vi "Equalize Channel.vi"(0 "input data":cdb[](array[numeric])=array[8192 elements], 7 "channel":T1) -> (3 "processing duration":dbl format="%#_6p", 4 "output data":cdb[](array[numeric]))   [LabVIEW 2019]
uses:
  3fdb30cd-5524-4ae9-8a8d-15974dc7fefb.vi
  <vilib>/Analysis/1siggen.llb/Ramp Pattern by Samples.vi
  <vilib>/Analysis/2dsp.llb/Complex FFT.vi
  <vilib>/Analysis/2dsp.llb/Inverse Complex FFT.vi
  e220b846-d6bb-41e5-8f9d-4ae727cf2950.vi
  <vilib>/Utility/High Resolution Relative Seconds.vi
  <vilib>/Utility/error.llb/Clear Errors.vi
  <vilib>/Analysis/NI_AALPro.lvlib
  <vilib>/Analysis/NI_AALBase.lvlib
  <vilib>/gmath/NI_Gmath.lvlib
panel:
  out "XY Graph":cluster{"xi used":dbl[], "yi":dbl[]}[](graph)
  out "XY Graph 2":cluster{"xi used":dbl[], "yi":dbl[]}(graph)
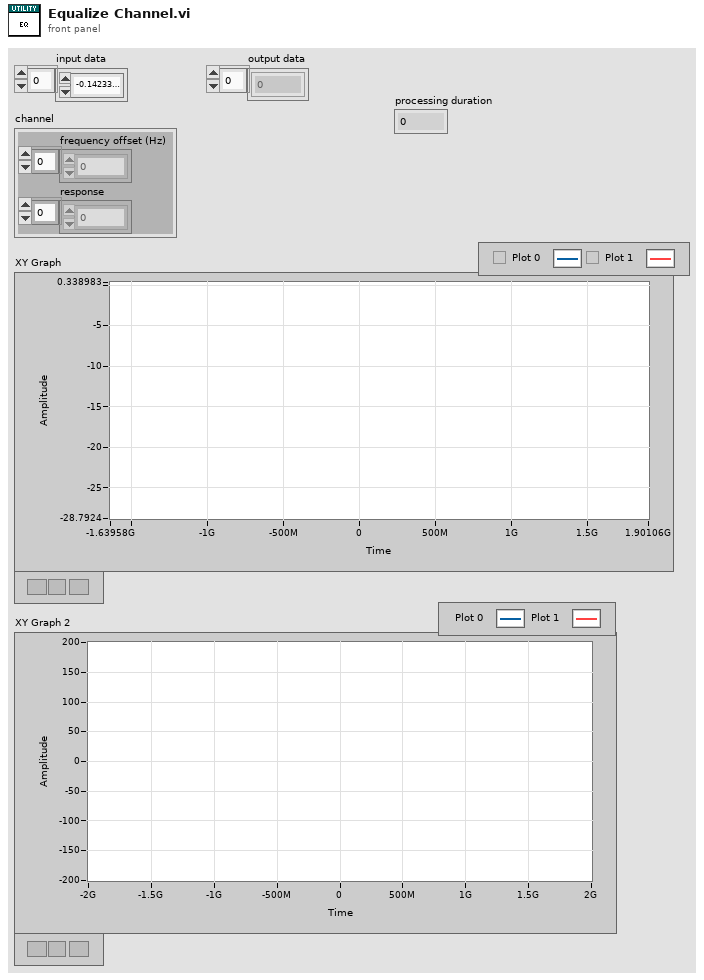
[diagram p1: front panel]
types:
  T1 = cluster{"frequency offset (Hz)":dbl[], "response":cdb[]}
  T2 = typedef "Constants.ctl" = cluster{"data clock rate (Hz)":dbl, "sample rate (Hz)":dbl, "sample rate selector string":string, "default tx bitfile path":path, "default rx bitfile path":path, "default proc bitfile path":path}
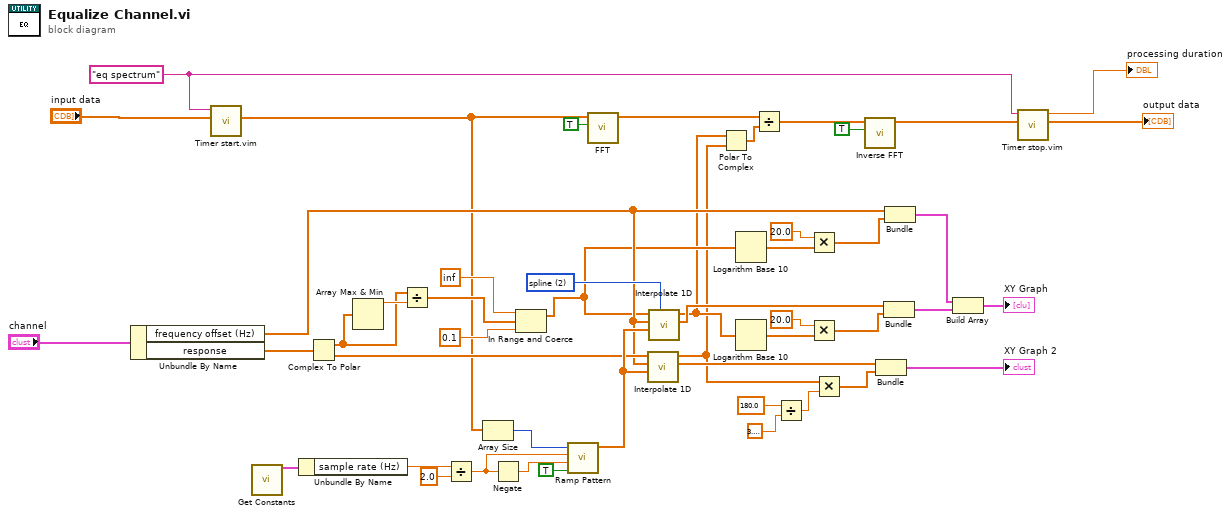
[diagram p0: block diagram]
diagram:
  w2 = "eq spectrum" ("timer name (t1)")
  w41 = 2 items=["nearest", "linear", "spline", "cubic Hermite", "Lagrange"] ("method")
  n1 = Unbundle By Name("channel") -> ("frequency offset (Hz)"=w27:dbl[], "response"=w29:cdb[])
  n2 = call "Timer start.vim"("dataflow in"="input data", "timer name (t1)"=w2) -> ("dataflow out"=w5:cdb[])  [unwired: 9 in]
  n3 = call "Get Constants.vi"() -> ("constants"=w8:T2)  [unwired: 15 in]
  n4 = Unbundle By Name(w8) -> ("sample rate (Hz)"=w7:dbl)
  n5 = Complex To Polar(r * e^(i*theta)=w29) -> (r=w25:dbl[], theta=w28:dbl[])
  n6 = Array Max & Min(array=w25) -> (max value=w26:dbl)  [unwired: 3 out]
  n7 = Divide(x=w25, y=w26) -> (x/y=w22:dbl[])
  n8 = Divide(x=w7, y=2.0) -> (x/y=w44:dbl)
  n9 = Array Size(array=w5) -> (size(s)=w42:i32)
  n10 = Negate(x=w44) -> (-x=w45:dbl)
  n11 = In Range and Coerce(upper limit=inf, x=w22, lower limit=0.1) -> (coerced(x)=w19:dbl[])  [unwired: 1 out]
  n12 = call-poly <vilib>:"Ramp Pattern.vi"("exclude end?"=TRUE, "start"=w45, "end"=w44, "samples"=w42) -> ("Ramp Pattern"=w40:dbl[])  [unwired: 6 in, 1 out]
  n13 = call-poly <vilib>:"FFT.vi"("shift?"=TRUE, "X"=w5) -> ("FFT {X}"=w31:cdb[])  [unwired: 8 in, 1 out]
  n14 = call <vilib>:"Interpolate 1D.vi"("xi"=w40, "X"=w27, "Y"=w28) -> ("xi used"=w35:dbl[], "yi"=w10:dbl[])  [unwired: 6 in, 1 out]
  n15 = call <vilib>:"Interpolate 1D.vi"("method"=w41, "xi"=w40, "X"=w27, "Y"=w19) -> ("xi used"=w39:dbl[], "yi"=w15:dbl[])  [unwired: 5 in, 1 out]
  n16 = Polar To Complex(1:w10, 2:w15) -> (0:w33:cdb[])
  n17 = Logarithm Base 10(1:w19) -> (0:w21:dbl[])
  n18 = Logarithm Base 10(1:w15) -> (0:w16:dbl[])
  n19 = Divide(x=w31, y=w33) -> (x/y=w30:cdb[])
  n20 = Divide(x=180.0, y=3.141592653589793) -> (x/y=w11:dbl)
  n21 = Multiply(x=20.0, y=w21) -> (x*y=w18:dbl[])
  n22 = Multiply(x=20.0, y=w16) -> (x*y=w14:dbl[])
  n23 = Multiply(x=w10, y=w11) -> (x*y=w9:dbl[])
  n24 = call-poly <vilib>:"Inverse FFT.vi"("shift?"=TRUE, "FFT {X}"=w30) -> ("X"=w4:cdb[])  [unwired: 8 in, 1 out]
  n25 = Bundle("xi used"=w35, w9) -> (→"XY Graph 2":cluster{"xi used":dbl[], dbl[]})  [unwired: 1 in]
  n26 = Bundle("xi used"=w39, w14) -> (w38:cluster{"xi used":dbl[], dbl[]})  [unwired: 1 in]
  n27 = Bundle("frequency offset (Hz)"=w27, w18) -> (w37:cluster{"frequency offset (Hz)":dbl[], dbl[]})  [unwired: 1 in]
  n28 = Build Array(w37, w38) -> (→"XY Graph":cluster{"xi used":dbl[], dbl[]}[])
  n29 = call "Timer stop.vim"("dataflow in"=w4, "timer name (t1)"=w2) -> ("dataflow out"=→"output data":cdb[], "final time"=→"processing duration":dbl)  [unwired: 8 in]
